vi "Process Triggers.vi"(1 "RT Data in":T1={"Device Ref"=18446744073709551615, "Waveforms"=[], "Channels"={"Command Chan Refs"=[], "Command Data Refs"=[], "Command Values"=[], "Status Chan Refs"=[], "Status Data Refs"=[], "Status Values"=[], "System Time"={"System Time"=timestamp(0 s since 1904-01-01), "Data Reference"=0, "Absolute Time Channel Data Ref"=0, "Get Date-Time Channel Data Ref"=0}, "Trigger Chan Refs"=[], "Trigger Data Refs"=[], "Trigger Values"=[]}, "Waveform Logs"=[], "Communication"={"Async Status"=refnum, "Wfm Comm Properties"={"WPL"={"Custom Queue Size"=1, "Use Custom Queue Size?"=FALSE}}, "Shutdown Event"=refnum, "Trigger Event"=refnum, "New File Event"=refnum, "Log Queues"=[], "Async VI Ref"=refnum}, "error"={"status"=FALSE, "code"=0, "source"=""}} {"Device Ref" format="%.0x"; "Channels"."Trigger Data Refs"."Data Reference" format="%.0x"; "Channels"."Trigger Chan Refs" format="%.0x"; "Channels"."System Time"."Get Date-Time Channel Data Ref" format="%.0x"; "Channels"."System Time"."Absolute Time Channel Data Ref" format="%.0x"; "Channels"."System Time"."Channel Data Reference" format="%.0x"; "Channels"."Status Data Refs"."Data Reference" format="%.0x"; "Channels"."Command Data Refs"."Data Reference" format="%.0x"; "Channels"."Status Chan Refs" format="%.0x"; "Channels"."Command Chan Refs" format="%.0x"; "Waveforms"."Waveform Ref in" format="%.0x"; "Waveform Logs"."Node ID" format="%.0x"; "Waveform Logs"."TDMS Error Code"."Data Ref" format="%.0x"; "Waveform Logs"."Missed Samples"."Data Ref" format="%.0x"; "Waveform Logs"."File Status"."Data Ref" format="%.0x"; "Waveform Logs"."Start New File"."Data Ref" format="%.0x"; "Waveform Logs"."Logging Enabled"."Data Ref" format="%.0x"; "Waveform Logs"."Stop Trigger"."Node Data Ref" format="%.0x"; "Waveform Logs"."Stop Trigger"."Node ID" format="%.0x"; "Waveform Logs"."Start Trigger"."Node Data Ref" format="%.0x"; "Waveform Logs"."Start Trigger"."Node ID" format="%.0x"}) -> (0 "RT Data out":T1={"Device Ref"=18446744073709551615, "Waveforms"=[], "Channels"={"Command Chan Refs"=[], "Command Data Refs"=[], "Command Values"=[], "Status Chan Refs"=[], "Status Data Refs"=[], "Status Values"=[], "System Time"={"System Time"=timestamp(0 s since 1904-01-01), "Data Reference"=0, "Absolute Time Channel Data Ref"=0, "Get Date-Time Channel Data Ref"=0}, "Trigger Chan Refs"=[], "Trigger Data Refs"=[], "Trigger Values"=[]}, "Waveform Logs"=[], "Communication"={"Async Status"=refnum, "Wfm Comm Properties"={"WPL"={"Custom Queue Size"=1, "Use Custom Queue Size?"=FALSE}}, "Shutdown Event"=refnum, "Trigger Event"=refnum, "New File Event"=refnum, "Log Queues"=[], "Async VI Ref"=refnum}, "error"={"status"=FALSE, "code"=0, "source"=""}} {"Device Ref" format="%.0x"; "Channels"."Trigger Data Refs"."Data Reference" format="%.0x"; "Channels"."Trigger Chan Refs" format="%.0x"; "Channels"."System Time"."Get Date-Time Channel Data Ref" format="%.0x"; "Channels"."System Time"."Absolute Time Channel Data Ref" format="%.0x"; "Channels"."System Time"."Channel Data Reference" format="%.0x"; "Channels"."Status Data Refs"."Data Reference" format="%.0x"; "Channels"."Command Data Refs"."Data Reference" format="%.0x"; "Channels"."Status Chan Refs" format="%.0x"; "Channels"."Command Chan Refs" format="%.0x"; "Waveforms"."Waveform Ref in" format="%.0x"; "Waveform Logs"."Node ID" format="%.0x"; "Waveform Logs"."TDMS Error Code"."Data Ref" format="%.0x"; "Waveform Logs"."Missed Samples"."Data Ref" format="%.0x"; "Waveform Logs"."File Status"."Data Ref" format="%.0x"; "Waveform Logs"."Start New File"."Data Ref" format="%.0x"; "Waveform Logs"."Logging Enabled"."Data Ref" format="%.0x"; "Waveform Logs"."Stop Trigger"."Node Data Ref" format="%.0x"; "Waveform Logs"."Stop Trigger"."Node ID" format="%.0x"; "Waveform Logs"."Start Trigger"."Node Data Ref" format="%.0x"; "Waveform Logs"."Start Trigger"."Node ID" format="%.0x"})   [LabVIEW 2015, in "Waveform Data Logger Engine.lvlib"]
uses:
  Waveform Data Logger Engine.lvlib
  Types/RT Data.ctl
  <vilib>/NI Veristand/Custom Device API/Custom Device Item Ref.ctl
  Types/Inline Waveform Info.ctl
  <vilib>/NI Veristand/Custom Device API/Waveform Data Reference.ctl
  Classes/Waveforms/Waveform Receive/Associated Log.ctl
  <vilib>/NI Veristand/Custom Device API/Custom Device Waveform DataType.ctl
  Types/Channels.ctl
  <vilib>/NI Veristand/Custom Device API/Block Data Reference.ctl
  <vilib>/NI Veristand/Custom Device API/Data Reference.ctl
  Types/System Time.ctl
  Types/Inline Waveform Log Info.ctl
  Classes/Log File Specifications/Waveform TDMS Log File Specification/Waveform TDMS Log File Specification.lvclass
  Classes/Triggers/Trigger/Trigger.lvclass
  Types/Inline Log Waveform.ctl
  Types/Trigger Settings.ctl
  Types/Log Status.ctl
  Types/Channel.ctl
  Types/Communication.ctl
  Types/Async Status.ctl
  Types/Async State.ctl
  <vilib>/NI Veristand/Custom Device Waveform API/Communication Properties.ctl
  Types/Trigger Event Data.ctl
  Types/Trigger Received.ctl
  Types/New File Event Data.ctl
  Types/Log Queues.ctl
  Classes/Triggers/Trigger/Trigger.lvclass/Trigger.ctl
  Classes/Triggers/Digital Edge Trigger/Digital Edge Trigger.lvclass/Digital Edge Trigger.ctl
  Classes/Triggers/Analog Edge Trigger/Analog Edge Trigger.lvclass/Analog Edge Trigger.ctl
  Classes/Triggers/Value Change Trigger/Value Change Trigger.lvclass/Value Change Trigger.ctl
  Classes/Triggers/Boolean Evaluation Trigger/Boolean Evaluation Trigger.lvclass/Boolean Evaluation Trigger.ctl
  Classes/Triggers/Default Trigger/Default Trigger.lvclass/Default Trigger.ctl
  Classes/Triggers/Trigger/Evaluate.vi
  Classes/Triggers/Trigger/Initialize.vi
  <vilib>/NI Veristand/Custom Device API/NI VeriStand - Get Channel Values by Block Data Reference.vi
  Classes/Triggers/Digital Edge Trigger/Evaluate Digital Edge Trigger.vi
  Classes/Triggers/Analog Edge Trigger/Evaluate Analog Edge Trigger.vi
  Classes/Triggers/Value Change Trigger/Evaluate Value Change Trigger.vi
  Classes/Triggers/Boolean Evaluation Trigger/Evaluate Boolean Evaluation Trigger.vi
  Classes/Triggers/Default Trigger/Evaluate Default Trigger.vi
  Classes/Triggers/Digital Edge Trigger/Initialize Digital Edge Trigger.vi
  Classes/Triggers/Analog Edge Trigger/Initialize Analog Edge Trigger.vi
  Classes/Triggers/Value Change Trigger/Initialize Value Change Trigger.vi
  Classes/Triggers/In Range Trigger/Evaluate In Range Trigger.vi
  <vilib>/NI Veristand/Custom Device API/Global Data Refs.vi
  Classes/Triggers/Default Trigger/Default Trigger.lvclass
  Classes/Triggers/In Range Trigger/In Range Trigger.lvclass
  Classes/Triggers/Boolean Evaluation Trigger/Boolean Evaluation Trigger.lvclass
  Classes/Triggers/Value Change Trigger/Value Change Trigger.lvclass
  Classes/Triggers/Analog Edge Trigger/Analog Edge Trigger.lvclass
  Classes/Triggers/Digital Edge Trigger/Digital Edge Trigger.lvclass
  <vilib>/NI Veristand/Custom Device API/Custom Device API.lvlib
  Classes/Waveforms/Waveform Receive/Waveform Receive.lvclass
  <vilib>/NI Veristand/Custom Device Waveform API/NI_VS Custom Device Waveform API.lvlib
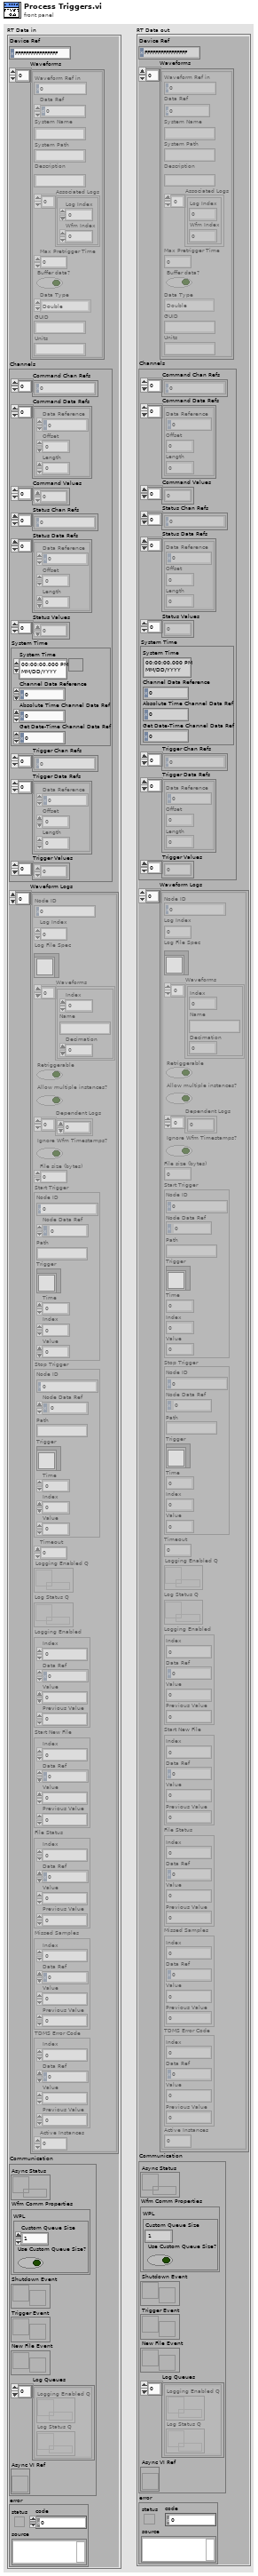
[diagram p1: front panel]
types:
  T1 = typedef "Waveform Data Logger Engine.lvlib/RT Data.ctl" = cluster{"Device Ref":T2, "Waveforms":T3[], "Channels":T7, "Waveform Logs":T11[], "Communication":T15, "error":errorcluster}
  T2 = typedef "Custom Device API.lvlib/Custom Device Item Ref.ctl" = u64
  T3 = typedef "Waveform Data Logger Engine.lvlib/Inline Waveform Info.ctl" = cluster{"Waveform Ref in":T2, "Data Ref":T4, "System Name":string, "System Path":string, "Description":string, "Associated Logs":T5[], "Max Pretrigger Time":dbl, "Buffer data?":bool, "Data Type":T6, "GUID":string, "Units":string}
  T4 = typedef "Custom Device API.lvlib/Waveform Data Reference.ctl" = i32
  T5 = typedef "Waveform Receive.lvclass/Associated Log.ctl" = cluster{"Log Index":i32, "Wfm Index":i32}
  T6 = typedef "Custom Device API.lvlib/Custom Device Waveform DataType.ctl" = enum16{"Double", "Complex Double"}
  T7 = typedef "Waveform Data Logger Engine.lvlib/Channels.ctl" = cluster{"Command Chan Refs":T2[], "Command Data Refs":T8[], "Command Values":dbl[], "Status Chan Refs":T2[], "Status Data Refs":T8[], "Status Values":dbl[], "System Time":T10, "Trigger Chan Refs":T2[], "Trigger Data Refs":T8[], "Trigger Values":dbl[]}
  T8 = typedef "Custom Device API.lvlib/Block Data Reference.ctl" = cluster{"Data Reference":T9, "Offset":u64, "Length":u64}
  T9 = typedef "Custom Device API.lvlib/Data Reference.ctl" = i32
  T10 = typedef "Waveform Data Logger Engine.lvlib/System Time.ctl" = cluster{"System Time":timestamp, "Data Reference":T9, "Absolute Time Channel Data Ref":T9, "Get Date-Time Channel Data Ref":T9}
  T11 = typedef "Waveform Data Logger Engine.lvlib/Inline Waveform Log Info.ctl" = cluster{"Node ID":T2, "Log Index":i32, "Log File Spec":refnum<class "Waveform TDMS Log File Specification.lvclass">, "Waveforms":T12[], "Retriggerable":bool, "Allow multiple instances?":bool, "Dependent Logs":i32[], "Ignore Wfm Timestamps?":bool, "File size (bytes)":i64, "Start Trigger":T13, "Stop Trigger":T13, "Timeout":dbl, "Logging Enabled Q":refnum<queue>, "Log Status Q":refnum<queue>, "Logging Enabled":T14, "Start New File":T14, "File Status":T14, "Missed Samples":T14, "TDMS Error Code":T14, "Active Instances":i32}
  T12 = typedef "Waveform Data Logger Engine.lvlib/Inline Log Waveform.ctl" = cluster{"Index":i32, "Name":string, "Decimation":u32}
  T13 = typedef "Waveform Data Logger Engine.lvlib/Trigger Settings.ctl" = cluster{"Node ID":T2, "Node Data Ref":i32, "Path":string, "Trigger":refnum<class "Trigger.lvclass">, "Time":dbl, "Index":i32, "Value":dbl}
  T14 = typedef "Waveform Data Logger Engine.lvlib/Channel.ctl" = cluster{"Index":i32, "Data Ref":T9, "Value":dbl, "Previous Value":dbl}
  T15 = typedef "Waveform Data Logger Engine.lvlib/Communication.ctl" = cluster{"Async Status":refnum<queue>, "Wfm Comm Properties":T16, "Shutdown Event":refnum<user-event>, "Trigger Event":refnum<user-event>, "New File Event":refnum<user-event>, "Log Queues":T17[], "Async VI Ref":refnum<vi>}
  T16 = typedef "NI_VS Custom Device Waveform API.lvlib/Communication Properties.ctl" = cluster{"WPL":cluster{"Custom Queue Size":i32, "Use Custom Queue Size?":bool}}
  T17 = typedef "Waveform Data Logger Engine.lvlib/Log Queues.ctl" = cluster{"Logging Enabled Q":refnum<queue>, "Log Status Q":refnum<queue>}
  T18 = typedef "Waveform Data Logger Engine.lvlib/Trigger Event Data.ctl" = cluster{"Log Index":i32, "Trigger Received":T19, "Start Trigger Time":timestamp, "Stop Trigger Time":timestamp}
  T19 = typedef "Waveform Data Logger Engine.lvlib/Trigger Received.ctl" = enum16{"None", "Start", "Stop", "Both", "Disable"}
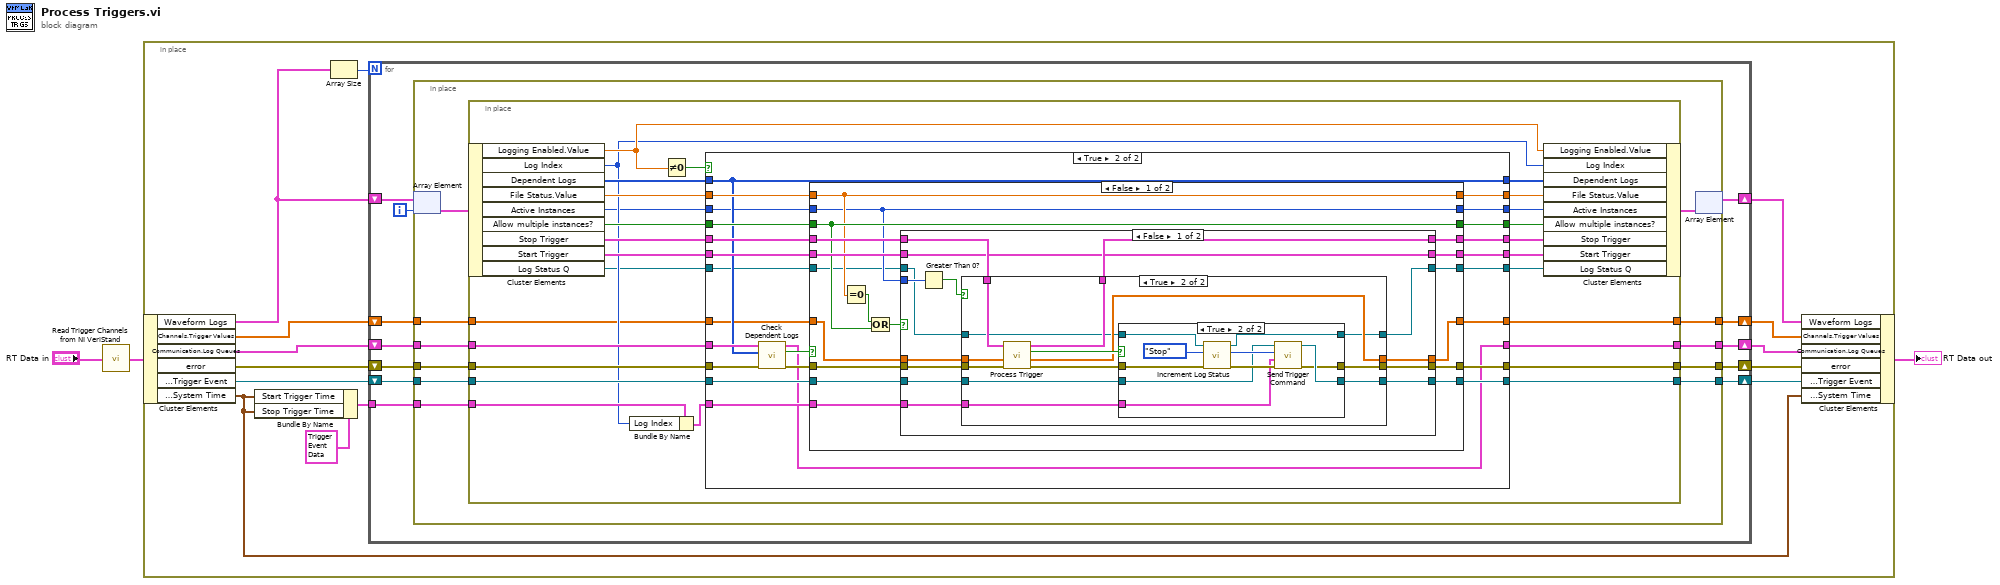
[diagram p0: block diagram]
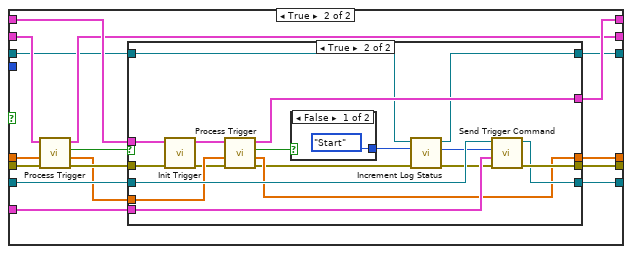
[diagram p5: hidden frame]
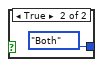
[diagram p7: hidden frame]
diagram:
  n1 = call "Read Trigger Channels from NI VeriStand.vi"("RT Data in"="RT Data in") -> ("RT Data out"=w1:T1)
  n2 = in-place {
    n3 = in-place-cluster #1(w1) -> ("Waveform Logs"=w9:T11[], "Channels.Trigger Values"=w5:dbl[], "Communication.Log Queues"=w12:T17[], "error"=w17:errorcluster, "Communication.Trigger Event"=w14:refnum<user-event>, "Channels.System Time.System Time"=w6:timestamp)
    n4 = Bundle By Name(cluster=T18 {"Log Index"=0, "Trigger Received"=enum."None", "Start Trigger Time"=timestamp(0 s since 1904-01-01), "Stop Trigger Time"=timestamp(0 s since 1904-01-01)} ("event data"), "Start Trigger Time"=w6, "Stop Trigger Time"=w6) -> (w10:T18)
    n5 = Array Size(array=w9) -> (size(s)=w16:i32)
    n6 = for {
      N: w16 -> [_]
      shift-right: [w23] -> w15
      shift-left: w17 -> [w29]
      shift-right: [w28] -> w8
      shift-left: w9 -> [w25]
      shift-right: [w21] -> w13
      shift-left: w14 -> [w27]
      shift-right: [w20] -> w7
      shift-left: w12 -> [w24]
      tunnel: w10 -> [w22]
      shift-right: [w18] -> w4
      shift-left: w5 -> [w19]
      i -> [w26]
      n7 = in-place {
        in-place-border: w29 -> [w38]
        in-place-border: w27 -> [w36]
        in-place-border: w24 -> [w39]
        in-place-border: [w37] -> w23
        in-place-border: w22 -> [w34]
        in-place-border: [w33] -> w21
        in-place-border: [w32] -> w20
        in-place-border: w19 -> [w31]
        in-place-border: [w30] -> w18
        n8 = in-place-array #2(w25, w26) -> (w40:T11)
        n9 = in-place {
          in-place-border: w39 -> [w66]
          in-place-border: w38 -> [w67]
          in-place-border: [w62] -> w37
          in-place-border: w36 -> [w64]
          in-place-border: w34 -> [w59]
          in-place-border: [w48] -> w33
          in-place-border: [w47] -> w32
          in-place-border: w31 -> [w44]
          in-place-border: [w43] -> w30
          n10 = in-place-cluster #3(w40) -> ("Logging Enabled.Value"=w50:dbl, "Log Index"=w49:i32, "Dependent Logs"=w52:i32[], "File Status.Value"=w56:dbl, "Active Instances"=w46:i32, "Allow multiple instances?"=w55:bool, "Stop Trigger"=w61:T13, "Start Trigger"=w60:T13, "Log Status Q"=w42:refnum<queue>)
          n11 = Bundle By Name(cluster=w59, "Log Index"=w49) -> (w63:T18)
          n12 = Not Equal To 0?(x=w50) -> (x != 0?=w65:bool)
          n13 = case shown="True" w65 {
            tunnel: w67 -> [w78 w102]
            tunnel: w52 -> [w75 w87]
            tunnel: w66 -> [w71 w101]
            tunnel: w56 -> [w74 w100]
            tunnel: w55 -> [w73 w99]
            tunnel: w60 -> [w76 w96]
            tunnel: w61 -> [w77 w95]
            tunnel: w64 -> [w72 w94]
            tunnel: w63 -> [_ w93]
            tunnel: [w78 w92] -> w62
            tunnel: [w77 w91] -> w58
            tunnel: [w76 w90] -> w57
            tunnel: [w74 w89] -> w54
            tunnel: [w73 w88] -> w53
            tunnel: [w75 w87] -> w51
            tunnel: [w72 w86] -> w48
            tunnel: [w71 w85] -> w47
            tunnel: w46 -> [w70 w84]
            tunnel: [w70 w83] -> w45
            tunnel: w44 -> [w69 w82]
            tunnel: [w69 w81] -> w43
            tunnel: w42 -> [w68 w80]
            tunnel: [w68 w79] -> w41
            frame False {
            }
            frame True {
              n14 = call "Check Dependent Logs.vi"("error in (no error)"=w102, "Dependent Logs"=w87, "Log Queues in"=w101) -> ("error out"=w97:errorcluster, "Active"=w98:bool, "Log Queues out"=w85:T17[])  [unwired: 6 in]
              n15 = case shown="False" w98 {
                tunnel: w100 -> [w109 w212]
                tunnel: w99 -> [w110 w211]
                tunnel: w97 -> [w117 w215]
                tunnel: w96 -> [w119 w213]
                tunnel: w95 -> [w118 w214]
                tunnel: w94 -> [w116 w210]
                tunnel: w93 -> [w115 _]
                tunnel: [w114 w215] -> w92
                tunnel: [w113 w214] -> w91
                tunnel: [w112 w213] -> w90
                tunnel: [w109 w212] -> w89
                tunnel: [w110 w211] -> w88
                tunnel: [w108 w210] -> w86
                tunnel: w84 -> [w107 w209]
                tunnel: [w107 w209] -> w83
                tunnel: w82 -> [w106 w208]
                tunnel: [w105 w208] -> w81
                tunnel: w80 -> [w104 w207]
                tunnel: [w103 w207] -> w79
                frame False {
                  n16 = Equal To 0?(x=w109) -> (x = 0?=w111:bool)
                  n17 = Or(x=w111, y=w110) -> (x .or. y?=w120:bool)
                  n18 = case shown="False" w120 {
                    tunnel: w119 -> [w128 w173]
                    tunnel: w118 -> [w134 w181]
                    tunnel: w117 -> [w133 w180]
                    tunnel: w116 -> [w132 w177]
                    tunnel: w115 -> [w131 w176]
                    tunnel: [w130 w175] -> w114
                    tunnel: [w129 w174] -> w113
                    tunnel: [w128 w172] -> w112
                    tunnel: [w127 w171] -> w108
                    tunnel: w107 -> [w126 _]
                    tunnel: w106 -> [w124 w170]
                    tunnel: [w123 w168] -> w105
                    tunnel: w104 -> [w122 w167]
                    tunnel: [w121 w166] -> w103
                    frame False {
                      n19 = Greater Than 0?(x=w126) -> (x > 0?=w125:bool)
                      n20 = case shown="True" w125 {
                        tunnel: w134 -> [w139 w152]
                        tunnel: w133 -> [w138 w151]
                        tunnel: w132 -> [w137 w149]
                        tunnel: w131 -> [_ w148]
                        tunnel: [w138 w146] -> w130
                        tunnel: [w139 w145] -> w129
                        tunnel: [w137 w144] -> w127
                        tunnel: w124 -> [w136 w143]
                        tunnel: [w136 w142] -> w123
                        tunnel: w122 -> [w135 w141]
                        tunnel: [w135 w140] -> w121
                        frame False {
                        }
                        frame True {
                          n21 = call "Process Trigger.vi"("error in (no error)"=w151, "Trigger Values in"=w143, "Trigger in"=w152) -> ("error out"=w147:errorcluster, "Trigger Values out"=w142:dbl[], "Trigger"=w150:bool, "Trigger out"=w145:T13)  [unwired: 5 in]
                          n22 = case shown="True" w150 {
                            tunnel: w149 -> [w154 w159]
                            tunnel: w148 -> [_ w156]
                            tunnel: w147 -> [w155 w165]
                            tunnel: [w155 w157] -> w146
                            tunnel: [w154 w158] -> w144
                            tunnel: w141 -> [w153 w163]
                            tunnel: [w153 w162] -> w140
                            frame False {
                            }
                            frame True {
                              n23 = call "Increment Log Status.vi"("error in"=w165, "Trigger Received in"=Trigger_Received."Stop" ("Trigger Received"), "Log Status Q in"=w163) -> ("error out"=w161:errorcluster, "Trigger Received out"=w160:T19, "Log Status Q out"=w162:refnum<queue>)  [unwired: 6 in]
                              n24 = call "Send Trigger Command.vi"("error in (no error)"=w161, "Trigger data"=w156, "Trigger Received in"=w160, "Trigger Event in"=w159) -> ("error out"=w157:errorcluster, "Trigger Event out"=w158:refnum<user-event>)  [unwired: 6 in]
                            }
                          }
                        }
                      }
                    }
                    frame True {
                      n25 = call "Process Trigger.vi"("error in (no error)"=w180, "Trigger Values in"=w170, "Trigger in"=w173) -> ("error out"=w179:errorcluster, "Trigger Values out"=w169:dbl[], "Trigger"=w178:bool, "Trigger out"=w172:T13)  [unwired: 5 in]
                      n26 = case shown="True" w178 {
                        tunnel: w179 -> [w186 w195]
                        tunnel: w181 -> [w185 w196]
                        tunnel: w177 -> [w184 w203]
                        tunnel: w176 -> [_ w202]
                        tunnel: [w186 w201] -> w175
                        tunnel: [w185 w200] -> w174
                        tunnel: [w184 w199] -> w171
                        tunnel: w169 -> [w183 w198]
                        tunnel: [w183 w197] -> w168
                        tunnel: w167 -> [w182 w188]
                        tunnel: [w182 w187] -> w166
                        frame False {
                        }
                        frame True {
                          n27 = call "Init Trigger.vi"("error in (no error)"=w195, "Trigger in"=w196) -> ("error out"=w194:errorcluster, "Trigger out"=w193:T13)  [unwired: 8 in]
                          n28 = call "Process Trigger.vi"("error in (no error)"=w194, "Trigger Values in"=w198, "Trigger in"=w193) -> ("error out"=w192:errorcluster, "Trigger Values out"=w197:dbl[], "Trigger"=w204:bool, "Trigger out"=w200:T13)  [unwired: 5 in]
                          n29 = case shown="False" w204 {
                            tunnel: [Trigger_Received."Start" ("Trigger Received") Trigger_Received."Both" ("Trigger Received")] -> w191
                            frame False {
                            }
                            frame True {
                            }
                          }
                          n30 = call "Increment Log Status.vi"("error in"=w192, "Trigger Received in"=w191, "Log Status Q in"=w188) -> ("error out"=w189:errorcluster, "Trigger Received out"=w190:T19, "Log Status Q out"=w187:refnum<queue>)  [unwired: 6 in]
                          n31 = call "Send Trigger Command.vi"("error in (no error)"=w189, "Trigger data"=w202, "Trigger Received in"=w190, "Trigger Event in"=w203) -> ("error out"=w201:errorcluster, "Trigger Event out"=w199:refnum<user-event>)  [unwired: 6 in]
                        }
                      }
                    }
                  }
                }
                frame True {
                }
              }
            }
          }
          n32 = in-place-cluster #3("Logging Enabled.Value"=w50, "Log Index"=w49, "Dependent Logs"=w51, "File Status.Value"=w54, "Active Instances"=w45, "Allow multiple instances?"=w53, "Stop Trigger"=w58, "Start Trigger"=w57, "Log Status Q"=w41) -> (w35:T11)
        }
        n33 = in-place-array #2(w35) -> (w28:T11[])  [unwired: 1 out]
      }
    }
    n34 = in-place-cluster #1("Waveform Logs"=w8, "Channels.Trigger Values"=w4, "Communication.Log Queues"=w7, "error"=w15, "Communication.Trigger Event"=w13, "Channels.System Time.System Time"=w6) -> (→"RT Data out":T1)
  }
